vi "Write Channel Names.vi"(8 "error in (no error)":errorcluster, 10 "Channel Names":string[](array[string]), 11 "Hardware Buzzer in":refnum<class "Hardware Buzzer.lvclass">) -> (0 "error out":errorcluster, 3 "Hardware Buzzer out":refnum<class "Hardware Buzzer.lvclass">)   [LabVIEW 2021, in "Hardware Buzzer.lvlib" / "Hardware Buzzer.lvclass"]
uses:
  Hardware Buzzer.lvclass
  Hardware Buzzer.lvclass/Hardware Buzzer.ctl
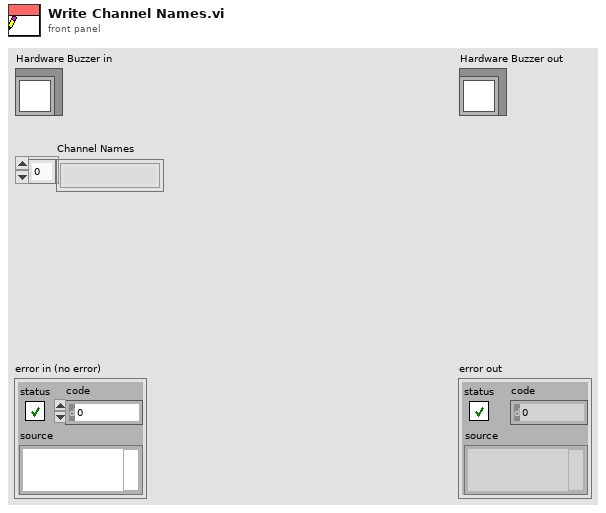
[diagram p1: front panel]
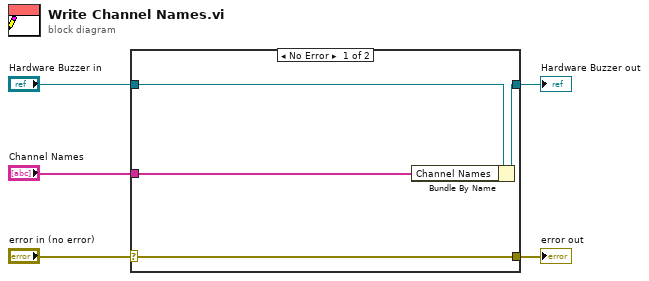
[diagram p0: block diagram]
diagram:
  n1 = case shown="No Error" "error in (no error)" {
    selector: "error in (no error)" -> [w9 w10]
    tunnel: [w9 w10] -> w4
    tunnel: [w7 w11] -> w2
    tunnel: "Hardware Buzzer in" -> [w8 w11]
    tunnel: "Channel Names" -> [w6 _]
    frame No Error {
      n2 = Bundle By Name(cluster=w8, "Channel Names"=w6) -> (w7:refnum<class "Hardware Buzzer.lvclass">)
    }
    frame Error {
    }
  }
  "error out" <- w4
  "Hardware Buzzer out" <- w2
